vi "hh.vi"() -> ()   [LabVIEW 2017]
uses:
  0fbf91d7-4518-4793-8bb0-b037e63db16a.vi
panel:
  out "Optitrack 2":string
  out "Cluster - Thin Border 2":T1
  in  "stop":bool
  out "String Indicator":string
  in  "Tab Control":T2(tab)
  in  "Settings Button":bool
  in  "Tools Button":bool
  in  "Function Selector":string(combo)
  out "String Indicator 2":string
  out "controls switch":T3
  in  "Back Button":bool
  in  "Forward Button":bool
  out "Boolean Rectangle":bool
  out "Boolean Rectangle 2":bool
  out "Boolean Rectangle 3":bool
  out "Boolean Rectangle 4":bool
  out "Boolean Rectangle 5":bool
  out "Boolean Rectangle 6":bool
  out "Boolean Rectangle 7":bool
  out "Boolean Rectangle 8":bool
  in  "Recording Path Selection":path
  in  "Back Button 3":bool
  in  "Forward Button 3":bool
  in  "Capture":bool
  out "Image Display":T4(plugin-control)
  out "String Indicator 3":string
  in  "Forward Button 2":bool
  in  "Back Button 2":bool
  # "Select Interior Color :-"
  # "Selected Interior Color :-"
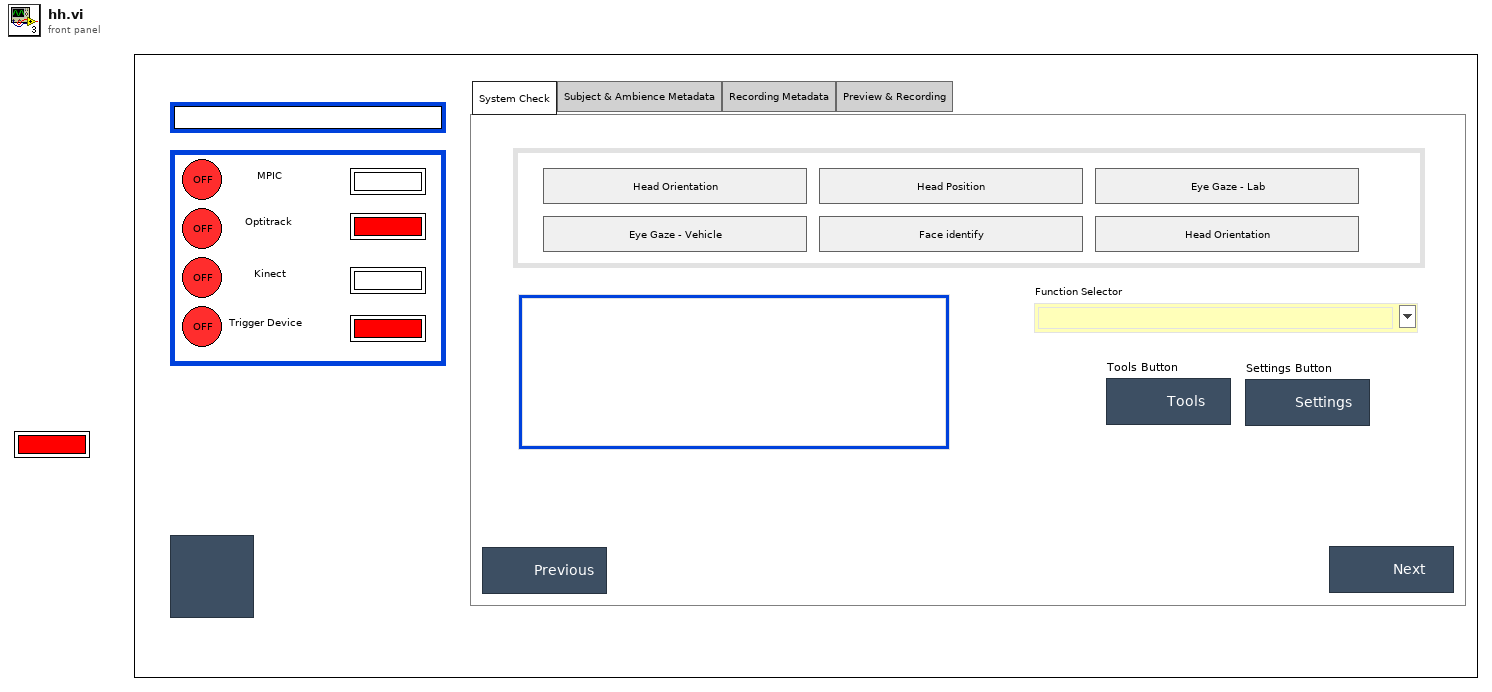
[diagram p1: front panel]
types:
  T1 = cluster{"MPIC":bool, "Optitrack":bool, "Kinect":bool, "Trigger Device":bool, "MPIC 2":string, "Optitrack 2":string, "Kinect 2":string, "Trigger Device 2":string}
  T2 = enum32{"System Check", "Subject & Ambience Metadata", "Recording Metadata", "Preview & Recording"}
  T3 = cluster{"Head Orientation":bool, "Head Orientation 2":bool, "Head Orientation 3":bool, "Head Orientation 4":bool, "Head Orientation 5":bool, "Head Orientation 6":bool}
  T4 = typedef "IMAQ Image.ctl" = refnum<image>
  T5 = cluster{"indicators":cluster{"MPIC":bool, "Optitrack":bool, "Kinect":bool, "Trigger Device":bool, "MPIC 2":string, "Optitrack 2":string, "Kinect 2":string, "Trigger Device 2":string}, "indicators value":cluster{"MPIC":bool, "Optitrack":bool, "Kinect":bool, "Trigger Device":bool, "MPIC 2":string, "Optitrack 2":string, "Kinect 2":string, "Trigger Device 2":string}[]}
  T6 = cluster{"MPIC":bool, "Optitrack":bool, "Kinect":bool, "Trigger Device":bool, "MPIC 2":string, "Optitrack 2":string, "Kinect 2":string, "Trigger Device 2":string}[]
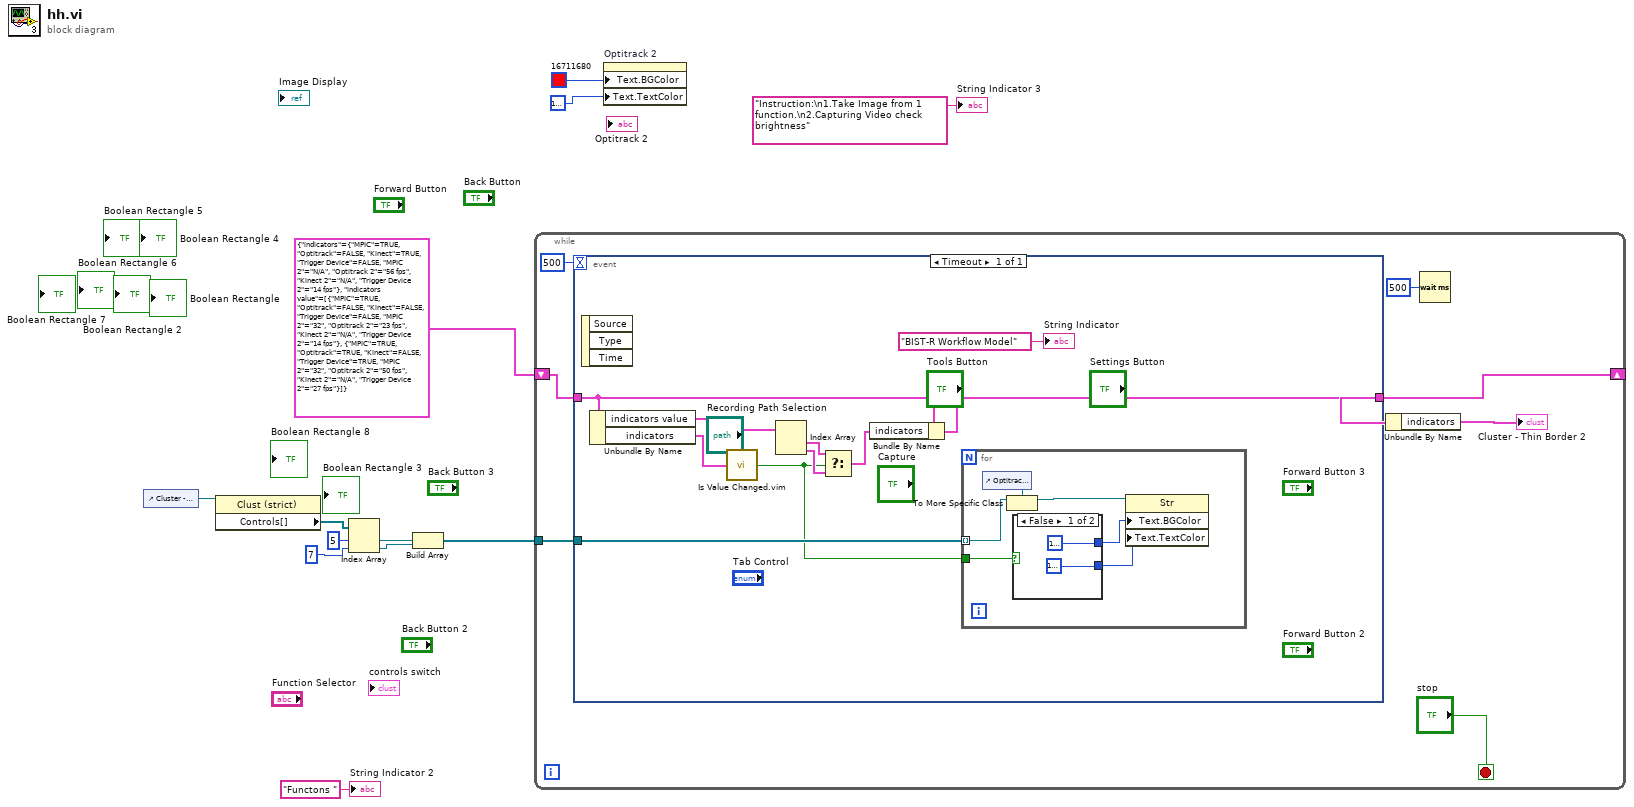
[diagram p0: block diagram]
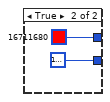
[diagram p2: hidden frame]
diagram:
  n1 = control-ref of="Cluster - Thin Border 2"() -> (w8:refnum<vi>)
  n2 = property on="Property Node" class="Clust (strict)"(reference=w8) -> ("Controls[]"=w7:refnum<vi>[])  [unwired: 1 in, 2 out]
  n3 = Index Array(array=w7, index #1=5 ("index"), index #2=7 ("index")) -> (element #1=w3:refnum<vi>, element #2=w4:refnum<vi>)
  n4 = Build Array(w3, w4) -> (w2:refnum<vi>[])
  n5 = while {
    shift-right: [w15] -> _
    shift-left: T5 {"indicators"={"MPIC"=TRUE, "Optitrack"=FALSE, "Kinect"=TRUE, "Trigger Device"=FALSE, "MPIC 2"="N/A", "Optitrack 2"="56 fps", "Kinect 2"="N/A", "Trigger Device 2"="14 fps"}, "indicators value"=[{"MPIC"=TRUE, "Optitrack"=FALSE, "Kinect"=FALSE, "Trigger Device"=FALSE, "MPIC 2"="32", "Optitrack 2"="23 fps", "Kinect 2"="N/A", "Trigger Device 2"="14 fps"}, {"MPIC"=TRUE, "Optitrack"=TRUE, "Kinect"=FALSE, "Trigger Device"=TRUE, "MPIC 2"="32", "Optitrack 2"="50 fps", "Kinect 2"="N/A", "Trigger Device 2"="27 fps"}]} -> [w16]
    tunnel: w2 -> [w13]
    stop <- "stop" stop-if-true
    n6 = event shown="[0] Timeout" {
      selector: _ -> [_]
      dyn-events: _ -> [_]
      timeout: 500 -> [_]
      tunnel: [w28] -> w15
      tunnel: w16 -> [w27]
      tunnel: w13 -> [w21]
      event Timeout {
        n7 = event-data() -> ()  [unwired: 1 in, 3 out]
        n8 = Unbundle By Name(w27) -> ("indicators value"=w26:T6, "indicators"=w22:T1)
        n9 = call "Is Value Changed.vim"("value"=w22) -> ("changed or first call?"=w20:bool)
        n10 = Index Array(array=w26) -> (element #1=w25:T1, element #2=w24:T1)  [unwired: 2 in]
        n11 = Select(t=w25, s=w20, f=w24) -> (s? t:f=w23:T1)
        n12 = Bundle By Name(cluster=w27, "indicators"=w23) -> (w28:T5)
        n13 = for {
          tunnel: w21 -> [w35] mode=indexing
          tunnel: w20 -> [w30]
          n14 = control-ref of="Optitrack 2"() -> (w33:refnum<vi>)
          n15 = To More Specific Class(target class=w33, reference=w35) -> (specific class reference=w34:refnum<vi>)  [unwired: 1 in, 1 out]
          n16 = case shown="False" w30 {
            tunnel: [u32 16777222 u32 16777226] -> w32
            tunnel: [u32 16777226 u32 16711680] -> w31
            frame False {
            }
            frame True {
            }
          }
          n17 = property on="Property Node" class="Str"(reference=w34, "Text.BGColor"=w31, "Text.TextColor"=w32) -> ()  [unwired: 1 in, 2 out]
        }
        "String Indicator" <- "BIST-R Workflow Model"
      }
    }
    n18 = Unbundle By Name(w15) -> ("indicators"=→"Cluster - Thin Border 2":T1)
    n19 = Wait (ms)(milliseconds to wait=u32 500) -> ()  [unwired: 1 out]
  }
  n20 = property on="Optitrack 2" class="Str"("Text.BGColor"=u32 16711680, "Text.TextColor"=u32 16777226) -> ()  [unwired: 2 in, 2 out]
  "String Indicator 2" <- "Functons " ("String Indicator 2")
  "String Indicator 3" <- "Instruction:\n1.Take Image from 1 function.\n2.Capturing Video check brightness" ("String Indicator 3")
